vi "Real PseudoInverse Matrix.vi"(2 "tolerance":dbl=-1.0 format="%.2f", 3 "Input Matrix":T1) -> (0 "error":i32, 1 "PseudoInverse Matrix":T1)   [LabVIEW 2020, in "NI_AALPro.lvlib"]
doc: "Finds the <B>PseudoInverse Matrix</B> of <B>Input Matrix</B>. Wire data to the <B>Input Matrix</B> input to determine the polymorphic instance to use or manually select the instance."
uses:
  NI_AALPro.lvlib
  RealMatrix.ctl
  <resource>/lvanlys.dll
  NI_Matrix.lvlib
panel:
  # "PseudoInverse Matrix"
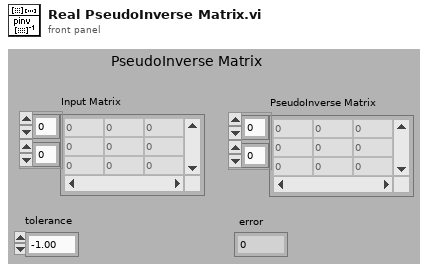
[diagram p1: front panel]
types:
  T1 = typedef "NI_Matrix.lvlib/RealMatrix.ctl" = dbl[][]
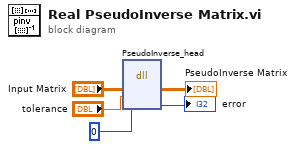
[diagram p0: block diagram]
diagram:
  n1 = dll-call lib="C:/Program Files (x86)/National Instruments/LabVIEW 2020/resource/lvanlys.*" fn="PseudoInverse_head"("Input Matrix"="Input Matrix", "tolerance"="tolerance", 0) -> ("Input Matrix"=→"PseudoInverse Matrix":T1, →"error":i32)  [unwired: 5 in, 2 out]
